vi "DataOut.vi"() -> ()   [LabVIEW 2013]
panel:
  out "Data Out":T1
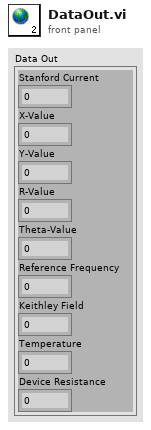
[diagram p1: front panel]
types:
  T1 = cluster{"Stanford Current":dbl, "X-Value":dbl, "Y-Value":dbl, "R-Value":dbl, "Theta-Value":dbl, "Reference Frequency":dbl, "Keithley Field":dbl, "Temperature":dbl, "Device Resistance":dbl}
diagram:
